vi "浊度_所有参数读取.vi"(8 "error in (no error)":errorcluster caption="错误输入（无错误）", 11 "MB session in":refnum<class "MB_Master.lvclass">) -> (0 "error out":errorcluster caption="错误输出", 2 "输出值":T1 {"电极型号标志" items=["NULL", "pH", "Cond", "DO", "Turb"]; "电极状态标志" items=["OK"=0, "第一点校正通过"=1, "第二点校正通过"=2, "悬浮物两点校准第一点校正通过"=11, "悬浮物两点校准第二点校正通过"=12, "浊度三点校正第一点校正通过"=31, "浊度三点校正第二点校正通过"=32, "浊度三点校正第三点校正通过"=33]}, 3 "MB session out":refnum<class "MB_Master.lvclass">)   [LabVIEW 2016, in "斯坦道多参数.lvlib"]
uses:
  <vilib>/Plasmionique/MB Master/MB_Master/MB_Master.lvclass
  <vilib>/Plasmionique/MB Master/MB Master.lvlib
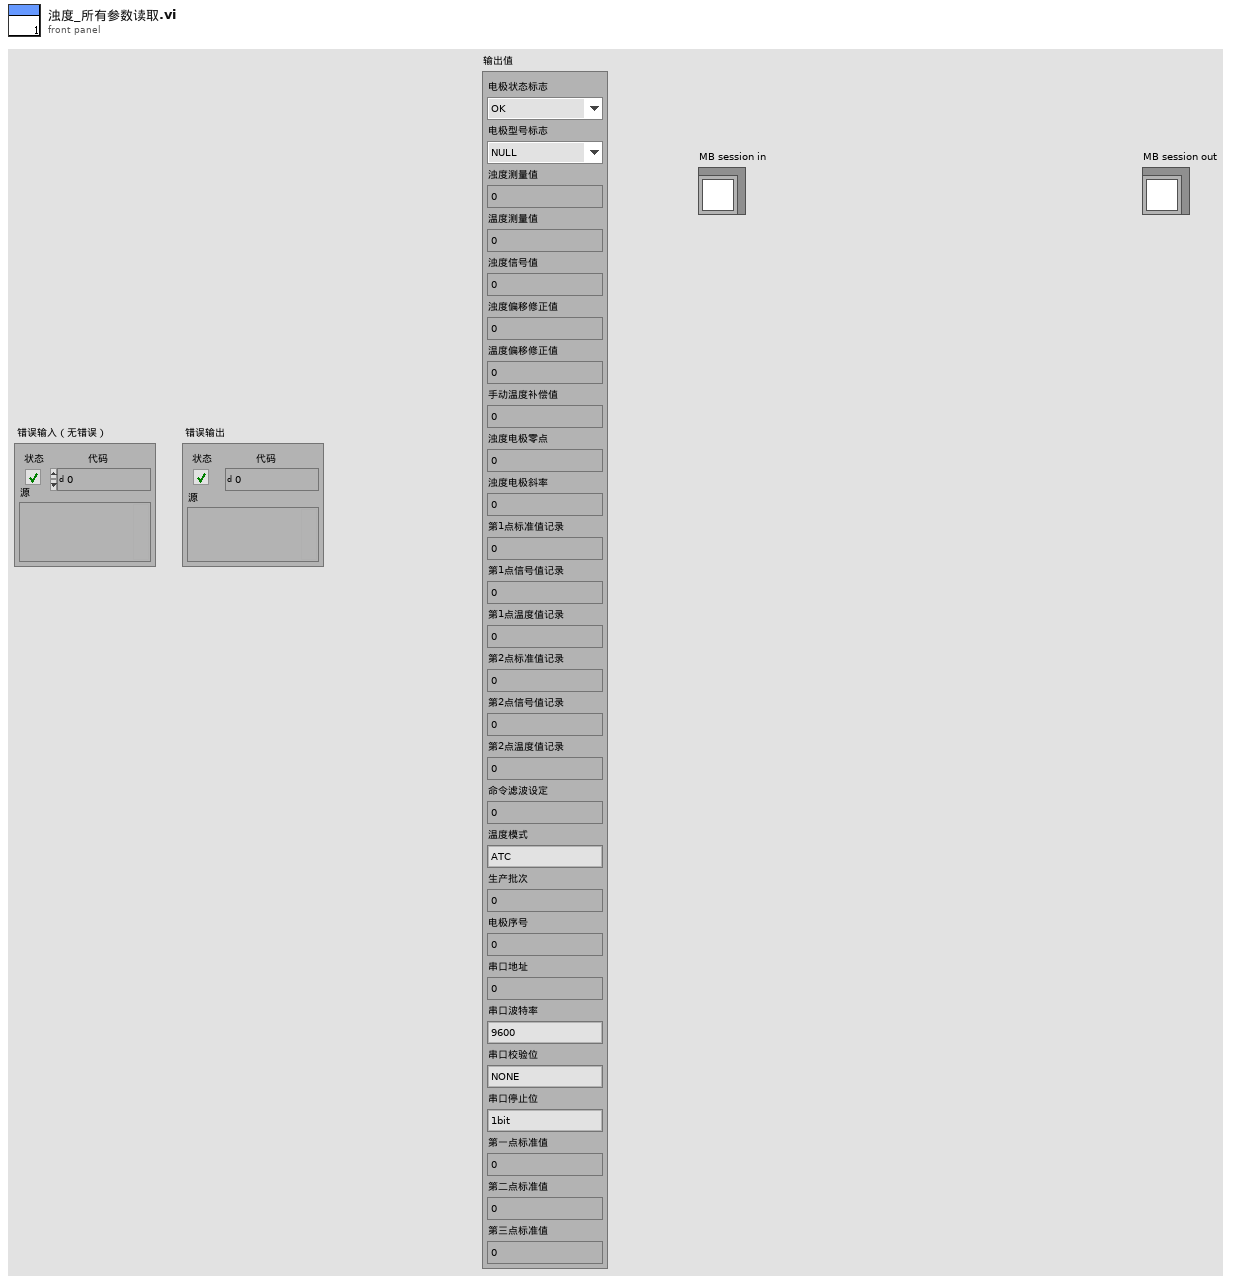
[diagram p1: front panel]
types:
  T1 = cluster{"电极状态标志":u16, "电极型号标志":u16, "浊度测量值":sgl, "温度测量值":sgl, "浊度信号值":sgl, "浊度偏移修正值":sgl, "温度偏移修正值":sgl, "手动温度补偿值":sgl, "浊度电极零点":sgl, "浊度电极斜率":sgl, "第1点标准值记录":sgl, "第1点信号值记录":sgl, "第1点温度值记录":sgl, "第2点标准值记录":sgl, "第2点信号值记录":sgl, "第2点温度值记录":sgl, "命令滤波设定":u16, "温度模式":enum16{"ATC", "MTC"}, "生产批次":u16, "电极序号":u16, "串口地址":u16, "串口波特率":enum16{"9600", "19200", "115200"}, "串口校验位":enum16{"NONE", "ODD", "EVEN"}, "串口停止位":enum16{"1bit", "2bit"}, "第一点标准值":sgl, "第二点标准值":sgl, "第三点标准值":sgl}
  T2 = cluster{u16, u16, "mode":dbl, "数值":sgl, "数值":sgl, "数值":sgl, "数值":sgl, "数值":sgl, "数值":sgl, "数值":sgl, "数值":sgl, "数值":sgl, "数值":sgl, "数值":sgl, "数值":sgl, "数值":sgl, u16, u16, u16, u16, u16, u16, u16, u16, "数值":sgl, "数值":sgl, "数值":sgl}
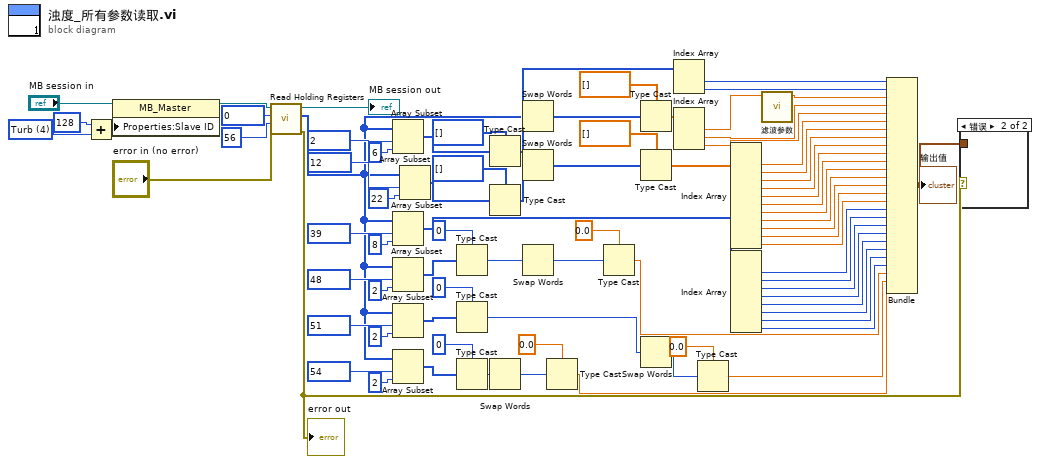
[diagram p0: block diagram]
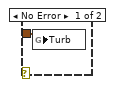
[diagram p2: hidden frame]
diagram:
  w80 = u16 4 items=["NULL", "pH", "Cond", "DO", "Turb"] ("数值")
  n1 = Add(x=u16 128, y=w80) -> (x+y=w79:u16)
  n2 = property class="MB_Master"(reference="MB session in", "Properties:Slave ID"=w79) -> (reference out=w16:refnum<class "MB_Master.lvclass">)  [unwired: 1 in, 1 out]
  n3 = call <vilib>:"Read Holding Registers.vi"("error in (no error)"="error in (no error)", "quantity"=u16 56, "starting address"=u16 0, "MB session in"=w16) -> ("error out"=w15:errorcluster, "Registers"=w6:u16[], "MB session out"=→"MB session out":refnum<class "MB_Master.lvclass">)  [unwired: 5 in]
  "error out" <- w15
  n4 = Array Subset(array=w6, index=u16 2 ("starting address"), length=6 ("长度")) -> (w68:u16[])
  n5 = Array Subset(array=w6, index=u16 39 ("starting address"), length=8 ("长度")) -> (w42:u16[])
  n6 = Array Subset(array=w6, index=u16 48 ("starting address"), length=2 ("长度")) -> (w25:u16[])
  n7 = Array Subset(array=w6, index=u16 51 ("starting address"), length=2 ("长度")) -> (w20:u16[])
  n8 = Array Subset(array=w6, index=u16 54 ("starting address"), length=2 ("长度")) -> (w13:u16[])
  n9 = Array Subset(array=w6, index=u16 12 ("starting address"), length=22 ("长度")) -> (w59:u16[])
  n10 = Type Cast(type=u32 0 ("数值"), x=w25) -> (*(type *) &x=w28:u32)
  n11 = Type Cast(type=u32 0 ("数值"), x=w20) -> (*(type *) &x=w22:u32)
  n12 = Type Cast(type=u32 0 ("数值"), x=w13) -> (*(type *) &x=w11:u32)
  n13 = Type Cast(type=u32[] [] ("数组 2"), x=w68) -> (*(type *) &x=w70:u32[])
  n14 = Type Cast(type=u32[] [] ("数组 2"), x=w59) -> (*(type *) &x=w62:u32[])
  n15 = Swap Words(1:w11) -> (0:w12:u32)
  n16 = Swap Words(1:w70) -> (0:w72:u32[])
  n17 = Swap Words(1:w62) -> (0:w63:u32[])
  n18 = Swap Words(1:w28) -> (0:w29:u32)
  n19 = Type Cast(type=sgl 0.0 ("数值"), x=w12) -> (*(type *) &x=w5:sgl)
  n20 = Type Cast(type=sgl 0.0 ("数值"), x=w29) -> (*(type *) &x=w19:sgl)
  n21 = Type Cast(type=sgl[] [] ("数组 2"), x=w72) -> (*(type *) &x=w67:sgl[])
  n22 = Type Cast(type=sgl[] [] ("数组 2"), x=w63) -> (*(type *) &x=w58:sgl[])
  n23 = Swap Words(1:w22) -> (0:w21:u32)
  n24 = Index Array(array=w6) -> (element #1=w75:u16, element #2=w74:u16)  [unwired: 2 in]
  n25 = Index Array(array=w67) -> (element #1=w2:sgl, element #2=w66:sgl, element #3=w65:sgl)  [unwired: 3 in]
  n26 = Type Cast(type=sgl 0.0 ("数值"), x=w21) -> (*(type *) &x=w18:sgl)
  n27 = Index Array(array=w58) -> (element #1=w57:sgl, element #2=w56:sgl, element #3=w55:sgl, element #4=w54:sgl, element #5=w53:sgl, element #6=w52:sgl, element #7=w51:sgl, element #8=w50:sgl, element #9=w49:sgl, element #10=w48:sgl, element #11=w47:sgl)  [unwired: 11 in]
  n28 = Index Array(array=w42) -> (element #1=w41:u16, element #2=w40:u16, element #3=w39:u16, element #4=w38:u16, element #5=w37:u16, element #6=w36:u16, element #7=w35:u16, element #8=w34:u16)  [unwired: 8 in]
  n29 = call "滤波参数.vi"("x"=w2) -> ("mode"=w1:dbl)  [unwired: 10 in]
  n30 = Bundle(w75, w74, "mode"=w1, "数值"=w66, "数值"=w65, "数值"=w57, "数值"=w56, "数值"=w55, "数值"=w54, "数值"=w53, "数值"=w52, "数值"=w51, "数值"=w50, "数值"=w49, "数值"=w48, "数值"=w47, w41, w40, w39, w38, w37, w36, w35, w34, "数值"=w19, "数值"=w18, "数值"=w5) -> (w14:T2)  [unwired: 1 in]
  "输出值" <- w14
  n31 = case shown="错误" w15 {
    tunnel: w14 -> [w81 _]
    frame No Error {
      n32 = global write "国弘过程全局变量.vi" "Turb"(w81) -> ()
    }
    frame Error {
    }
  }
